vi "stim config array to description array (subVI).vi"(8 "add duration? (F)":bool, 9 "add index? (F)":bool, 10 "stim. config array":T1 {"right odor"."port-odor ring" items=["off"]; "middle odor"."port-odor ring" items=["off"]; "left odor"."port-odor ring" items=["off"]}) -> (2 "description []":string[](array[string]))   [LabVIEW 2021]
uses:
  type-defs/stimulation configuration array (type def).ctl
  type-defs/stimulator configuration line cluster (type def).ctl
  type-defs/port-odor with color cluster (type def).ctl
  type-defs/port-odor ring (type def).ctl
  type-defs/odor color (type def).ctl
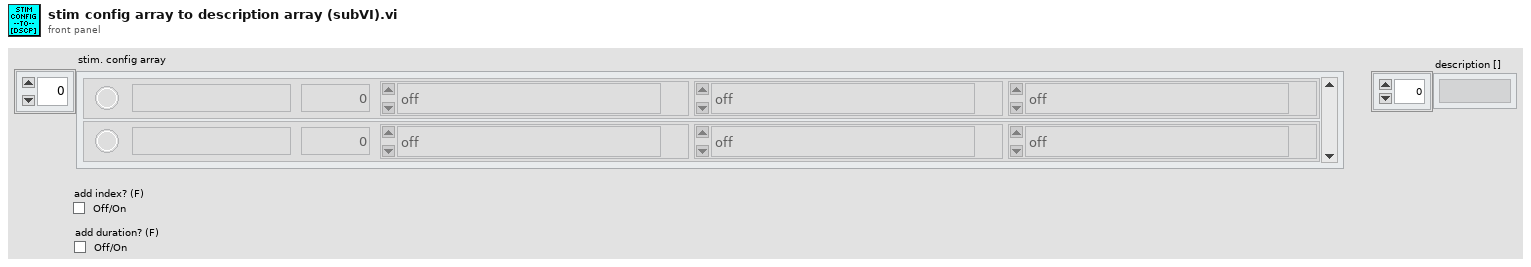
[diagram p1: front panel]
types:
  T1 = typedef "stimulation configuration array (type def).ctl" = T2[]
  T2 = typedef "stimulator configuration line cluster (type def).ctl" = cluster{"description":string, "duration, s":dbl, "left odor":T3, "middle odor":T3, "right odor":T3, "selected?":bool}
  T3 = typedef "port-odor with color cluster (type def).ctl" = cluster{"port-odor ring":T4, "odor color":T5}
  T4 = typedef "port-odor ring (type def).ctl" = u16
  T5 = typedef "odor color (type def).ctl" = u16
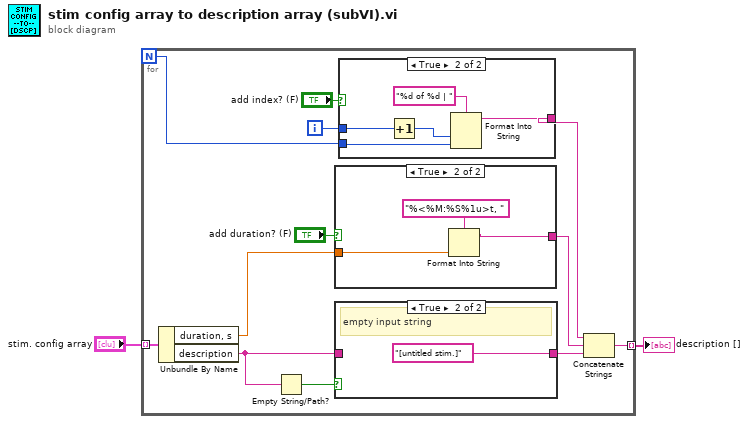
[diagram p0: block diagram]
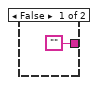
[diagram p3: hidden frame]
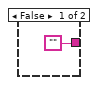
[diagram p4: hidden frame]
diagram:
  n1 = for {
    N -> [w10]
    tunnel: "stim. config array" -> [w14] mode=indexing
    tunnel: [w8] -> w1 mode=indexing
    i -> [w11]
    n2 = Unbundle By Name(w14) -> ("duration, s"=w5:dbl, "description"=w12:string)
    n3 = Empty String/Path?(string/path=w12) -> (empty?=w13:bool)
    n4 = case shown="True" "add duration? (F)" {
      tunnel: w5 -> [_ w20]
      tunnel: ["" w18] -> w3
      frame False {
      }
      frame True {
        n5 = Format Into String(format string="%<%M:%S%1u>t, ", w20) -> (resulting string=w18:string)  [unwired: 2 in, 1 out]
      }
    }
    n6 = case shown="True" w13 {
      tunnel: [w15 "[untitled stim.]" ("format string")] -> w9
      tunnel: w12 -> [w15 _]
      frame False {
        # "non-empty input"
      }
      frame True {
        # "empty input string"
      }
    }
    n7 = case shown="True" "add index? (F)" {
      tunnel: w11 -> [_ w25]
      tunnel: w10 -> [_ w23]
      tunnel: ["" w22] -> w4
      frame False {
      }
      frame True {
        n8 = Increment(x=w25) -> (x+1=w26:i32)
        n9 = Format Into String(format string="%d of %d | ", w26, w23) -> (resulting string=w22:string)  [unwired: 2 in, 1 out]
      }
    }
    n10 = Concatenate Strings(w4, w3, w9) -> (w8:string)
  }
  "description []" <- w1
